vi "AVERage.vi"(8 "Error in (no error)":errorcluster, 9 "Count":u16, 10 "Function":enum16{"AVERage:COUNt query", "AVERage:COUNt"}(ring), 11 "VISA resource":refnum<visa-resource-name>) -> (0 "Error out":errorcluster, 2 "Count out":u16, 3 "Dup VISA resource":refnum<visa-resource-name>)   [LabVIEW 2010]
doc: "Copyright (c) 2012 Metrolab Technology SA, Plan-les-Ouates, Geneva, Switzerland\nSet or retrieve the averaging count."
panel:
  # "AVERage"
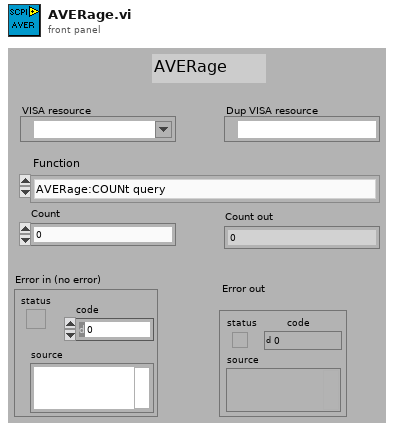
[diagram p1: front panel]
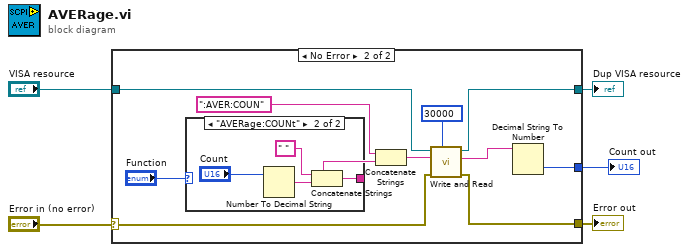
[diagram p0: block diagram]
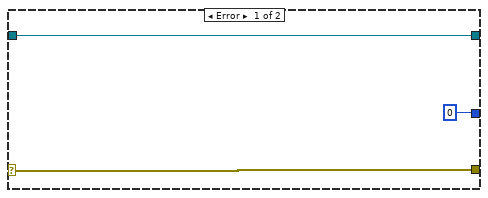
[diagram p2: hidden frame]
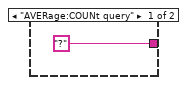
[diagram p3: hidden frame]
diagram:
  n1 = case shown="No Error" "Error in (no error)" {
    selector: "Error in (no error)" -> [w8 w17]
    tunnel: [w8 w16] -> w5
    tunnel: [w7 w12] -> w3
    tunnel: "VISA resource" -> [w7 w11]
    tunnel: [0 ("offset past number") w9] -> w1
    frame Error {
    }
    frame No Error {
      n2 = case shown="\"AVERage:COUNt\"" "Function" {
        tunnel: ["?" w21] -> w13
        frame "AVERage:COUNt query" {
        }
        frame "AVERage:COUNt" {
          n3 = Number To Decimal String(number="Count") -> (decimal integer string=w22:string)  [unwired: 1 in]
          n4 = Concatenate Strings(" " ("string"), w22) -> (w21:string)
        }
      }
      n5 = Concatenate Strings(":AVER:COUN", w13) -> (w18:string)
      n6 = call "Write and Read.vi"("Timeout (ms)"=u32 30000, "Error in (no error)"=w17, "Command"=w18, "VISA resource"=w11) -> ("Error out"=w16:errorcluster, "Response"=w10:string, "Dup VISA resource"=w12:refnum<visa-resource-name>)  [unwired: 3 in, 2 out]
      n7 = Decimal String To Number(string=w10) -> (number=w9:i32)  [unwired: 2 in, 1 out]
    }
  }
  "Error out" <- w5
  "Dup VISA resource" <- w3
  "Count out" <- w1
